vi "Read Ranges.vi"(8 "error in (no error)":errorcluster, 11 "FormulaG API in":refnum<class "FormulaG API.lvclass">) -> (0 "error out":errorcluster, 2 "Ranges":T1, 3 "FormulaG API out":refnum<class "FormulaG API.lvclass">)   [LabVIEW 2020]
uses:
  FormulaG API.lvclass
  Command.ctl
  FormulaG-Common/Ranges.ctl
  FormulaG-Common/FormulaG-Common.lvlib
  <vilib>/IlluminatedG/IG GodotServer/GodotLV/GodotServer/GodotServer.lvclass
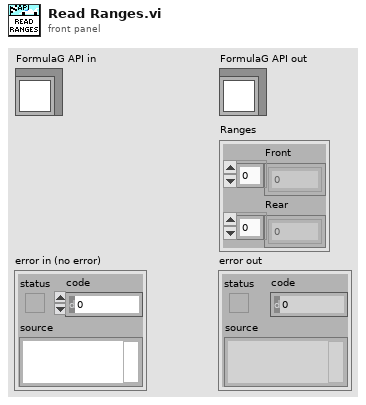
[diagram p1: front panel]
types:
  T1 = typedef "FormulaG-Common.lvlib/Ranges.ctl" = cluster{"Front":sgl[], "Rear":sgl[]}
  T2 = enum16{"big-endian, network order", "native, host order", "little-endian"}
  T3 = typedef "FormulaG.lvlib/FormulaG API.lvclass/Command.ctl" = enum8{"None", "Reset Car", "Request State", "Control Car", "Request Info", "Set Options", "Set Camera", "Set Pause", "Request Time"}
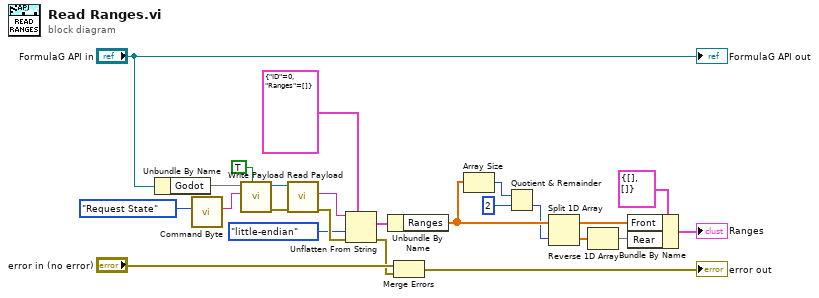
[diagram p0: block diagram]
diagram:
  n1 = Unbundle By Name("FormulaG API in") -> ("Godot"=w17)
  n2 = call "Command Byte.vi"("Command"=Command."Request State") -> ("Command Byte"=w16:string)  [unwired: 10 in]
  n3 = call <vilib>:"Write Payload.vi"("Binary (F = Text)"=TRUE, "Payload"=w16, "GodotServer in"=w17) -> ("error out"=w13:errorcluster, "GodotServer out"=w20:refnum<class "GodotServer.lvclass">)  [unwired: 7 in]
  n4 = call <vilib>:"Read Payload.vi"("error in (no error)"=w13, "GodotServer in"=w20) -> ("error out"=w24:errorcluster, "Payload"=w19:string)  [unwired: 7 in, 1 out]
  n5 = Unflatten From String(type=cluster{"ID":u8, "Ranges":sgl[]} {"ID"=0, "Ranges"=[]}, binary string=w19, byte order (0:big-endian, network order)=T2."little-endian", error in (no error)=w24) -> (value=w14:cluster{"ID":u8, "Ranges":sgl[]}, error out=w7:errorcluster)  [unwired: 1 in, 1 out]
  n6 = Unbundle By Name(w14) -> ("Ranges"=w10:sgl[])
  n7 = Merge Errors("error in (no error)", w7) -> (→"error out":errorcluster)
  n8 = Array Size(array=w10) -> (size(s)=w12:i32)
  n9 = Quotient & Remainder(x=w12, y=2) -> (floor(x/y)=w9:i32)  [unwired: 1 out]
  n10 = Split 1D Array(array=w10, index=w9) -> (first subarray=w3:sgl[], second subarray=w4:sgl[])
  n11 = Reverse 1D Array(array=w4) -> (reversed array=w2:sgl[])
  n12 = Bundle By Name(cluster=T1 {"Front"=[], "Rear"=[]} ("Ranges"), "Front"=w3, "Rear"=w2) -> (→"Ranges":T1)
  "FormulaG API out" <- "FormulaG API in"
